vi "Create1.vi"(8 "error in (no error)":errorcluster) -> (0 "error out":errorcluster, 2 "Model":refnum<class "3D Object.lvclass">, 3 "Level out":refnum<class "Level.lvclass">)   [LabVIEW 2015, in "Level.lvclass"]
uses:
  Level.lvclass
  3D Object/3D Object.lvclass
  Segment.ctl
  Point.ctl
  Level.lvclass/Level.ctl
  3D Object/Object.vi
  3D Object/Box.vi
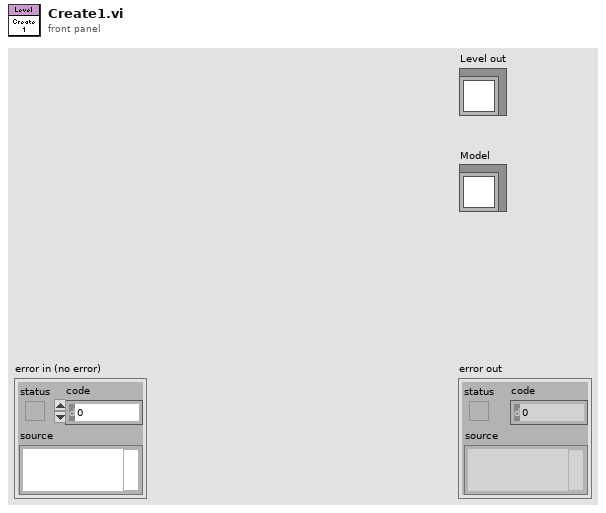
[diagram p1: front panel]
types:
  T1 = enum16{"As a Decal", "With Modulation", "With Blending", "As a replacement"}
  T2 = enum16{"No Filtration", "Linear Filtration", "Simple Mipmap Filtration", "Bilinear Filtration", "Trilinear Filtration"}
  T3 = cluster{"MinX":sgl, "MaxX":sgl, "MinZ":sgl, "MaxZ":sgl, "MinY":sgl, "MaxY":sgl}
  T4 = cluster{"Length X":sgl, "Length Y":sgl, "Length Z":sgl}
  T5 = typedef "Level.lvclass/Segment.ctl" = cluster{"Point 1":T6, "Point 2":T6}
  T6 = typedef "Level.lvclass/Point.ctl" = cluster{"Z":dbl, "X":dbl}
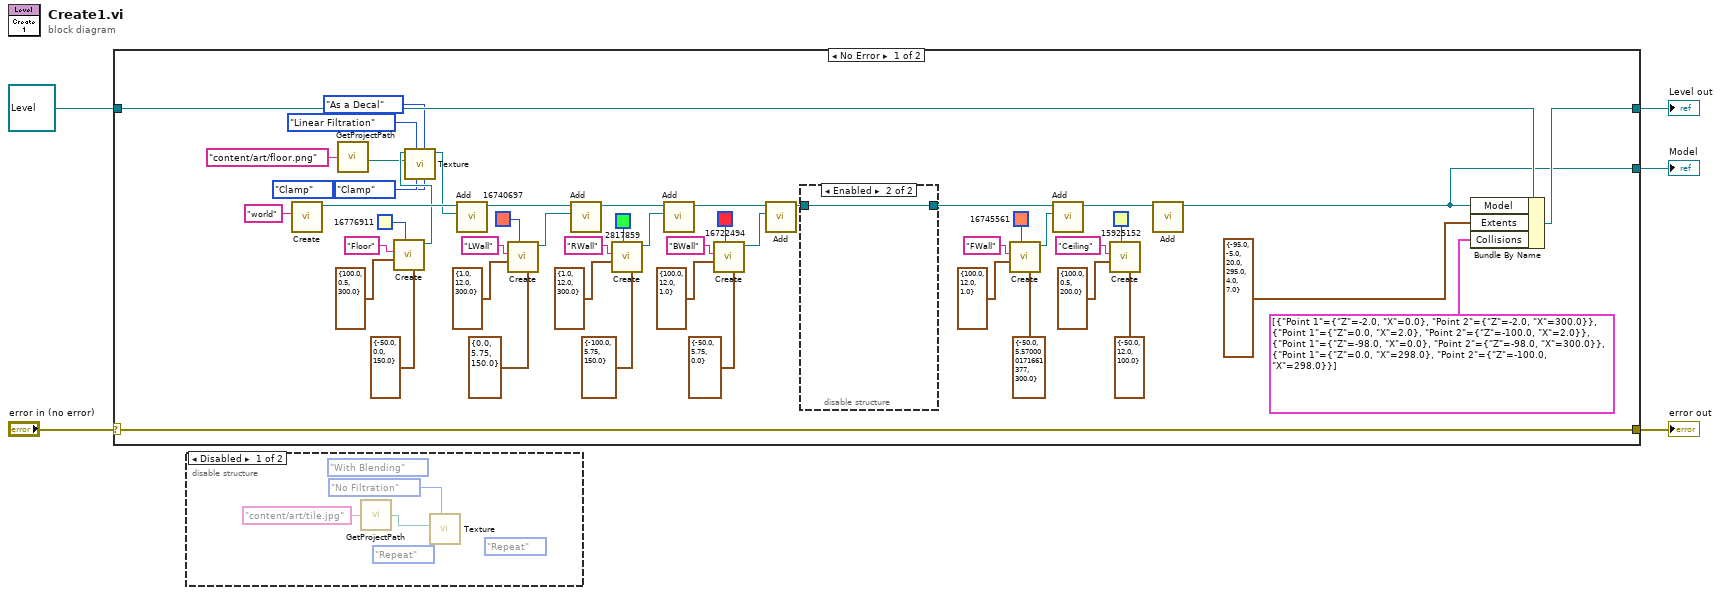
[diagram p0: block diagram]
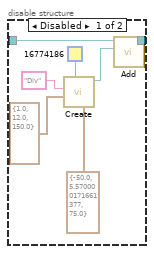
[diagram p3: hidden frame]
diagram:
  n1 = case shown="No Error" "error in (no error)" {
    selector: "error in (no error)" -> [w55 w65]
    tunnel: [w55 w65] -> w4
    tunnel: [w51 w64] -> w2
    tunnel: refnum<class "Level.lvclass"> refnum ("Level in") -> [w52 w64]
    tunnel: [w16 _] -> w1
    frame No Error {
      n2 = call-poly "Create.vi"("Name"="world") -> ("3D Object out"=w17:refnum<class "3D Object.lvclass">)  [unwired: 9 in, 1 out]
      n3 = call "GetProjectPath.vi"("File"="content/art/floor.png") -> ("Path"=w14:path)
      n4 = call-poly "Create.vi"("Position"=cluster{"X":sgl, "Y":sgl, "Z":sgl} {"X"=-50.0, "Y"=0.0, "Z"=150.0}, "Color Box"=u32 16776911, "Size"=T4 {"Length X"=100.0, "Length Y"=0.5, "Length Z"=300.0}, "Name"="Floor") -> ("3D Object out"=w15:refnum<class "3D Object.lvclass">)  [unwired: 6 in, 1 out]
      n5 = call "Texture.vi"("Vertical Wrap Mode"=enum16{"Clamp", "Repeat"}."Clamp", "Apply Mode"=T1."As a Decal", "Horizontal Wrap Mode"=enum16{"Clamp", "Repeat"}."Clamp", "Filter Mode"=T2."Linear Filtration", "path to image"=w14, "Object in"=w15) -> ("Object out"=w8:refnum<class "3D Object.lvclass">)  [unwired: 4 in, 1 out]
      n6 = call "Add.vi"("Child in"=w8, "Parent in"=w17) -> ("Parent out"=w18:refnum<class "3D Object.lvclass">)  [unwired: 7 in, 2 out]
      n7 = call-poly "Create.vi"("Position"=cluster{"X":sgl, "Y":sgl, "Z":sgl} {"X"=0.0, "Y"=5.75, "Z"=150.0}, "Color Box"=u32 16740697, "Size"=T4 {"Length X"=1.0, "Length Y"=12.0, "Length Z"=300.0}, "Name"="LWall") -> ("3D Object out"=w45:refnum<class "3D Object.lvclass">)  [unwired: 6 in, 1 out]
      n8 = call "Add.vi"("Child in"=w45, "Parent in"=w18) -> ("Parent out"=w44:refnum<class "3D Object.lvclass">)  [unwired: 7 in, 2 out]
      n9 = call-poly "Create.vi"("Position"=cluster{"X":sgl, "Y":sgl, "Z":sgl} {"X"=-100.0, "Y"=5.75, "Z"=150.0}, "Color Box"=u32 2817859, "Size"=T4 {"Length X"=1.0, "Length Y"=12.0, "Length Z"=300.0}, "Name"="RWall") -> ("3D Object out"=w43:refnum<class "3D Object.lvclass">)  [unwired: 6 in, 1 out]
      n10 = call "Add.vi"("Child in"=w43, "Parent in"=w44) -> ("Parent out"=w40:refnum<class "3D Object.lvclass">)  [unwired: 7 in, 2 out]
      n11 = call-poly "Create.vi"("Position"=cluster{"X":sgl, "Y":sgl, "Z":sgl} {"X"=-50.0, "Y"=5.75, "Z"=0.0}, "Color Box"=u32 16722494, "Size"=T4 {"Length X"=100.0, "Length Y"=12.0, "Length Z"=1.0}, "Name"="BWall") -> ("3D Object out"=w7:refnum<class "3D Object.lvclass">)  [unwired: 6 in, 1 out]
      n12 = call "Add.vi"("Child in"=w7, "Parent in"=w40) -> ("Parent out"=w34:refnum<class "3D Object.lvclass">)  [unwired: 7 in, 2 out]
      n13 = disable-structure shown="Enabled" {
        disable-tunnel: w34 -> [w62 w63]
        disable-tunnel: [w57 w63] -> w27
        frame Disabled {
          n14 = call-poly "Create.vi"("Position"=cluster{"X":sgl, "Y":sgl, "Z":sgl} {"X"=-50.0, "Y"=5.57, "Z"=75.0}, "Color Box"=u32 16774186, "Size"=T4 {"Length X"=1.0, "Length Y"=12.0, "Length Z"=150.0}, "Name"="Div") -> ("3D Object out"=w61:refnum<class "3D Object.lvclass">)  [unwired: 6 in, 1 out]
          n15 = call "Add.vi"("Child in"=w61, "Parent in"=w62) -> ("Parent out"=w57:refnum<class "3D Object.lvclass">)  [unwired: 7 in, 2 out]
        }
        frame Enabled {
        }
      }
      n16 = call-poly "Create.vi"("Position"=cluster{"X":sgl, "Y":sgl, "Z":sgl} {"X"=-50.0, "Y"=5.57, "Z"=300.0}, "Color Box"=u32 16745561, "Size"=T4 {"Length X"=100.0, "Length Y"=12.0, "Length Z"=1.0}, "Name"="FWall") -> ("3D Object out"=w6:refnum<class "3D Object.lvclass">)  [unwired: 6 in, 1 out]
      n17 = call "Add.vi"("Child in"=w6, "Parent in"=w27) -> ("Parent out"=w26:refnum<class "3D Object.lvclass">)  [unwired: 7 in, 2 out]
      n18 = call-poly "Create.vi"("Position"=cluster{"X":sgl, "Y":sgl, "Z":sgl} {"X"=-50.0, "Y"=12.0, "Z"=100.0}, "Color Box"=u32 15925152, "Size"=T4 {"Length X"=100.0, "Length Y"=0.5, "Length Z"=200.0}, "Name"="Ceiling") -> ()  [unwired: 6 in, 2 out]
      n19 = call "Add.vi"("Parent in"=w26) -> ("Parent out"=w16:refnum<class "3D Object.lvclass">)  [unwired: 8 in, 2 out]
      n20 = Bundle By Name(cluster=w52, "Model"=w16, "Extents"=T3 {"MinX"=-95.0, "MaxX"=-5.0, "MinZ"=20.0, "MaxZ"=295.0, "MinY"=4.0, "MaxY"=7.0}, "Collisions"=T5[] [{"Point 1"={"Z"=-2.0, "X"=0.0}, "Point 2"={"Z"=-2.0, "X"=300.0}}, {"Point 1"={"Z"=0.0, "X"=2.0}, "Point 2"={"Z"=-100.0, "X"=2.0}}, {"Point 1"={"Z"=-98.0, "X"=0.0}, "Point 2"={"Z"=-98.0, "X"=300.0}}, {"Point 1"={"Z"=0.0, "X"=298.0}, "Point 2"={"Z"=-100.0, "X"=298.0}}]) -> (w51:refnum<class "Level.lvclass">)
    }
    frame Error {
    }
  }
  "error out" <- w4
  "Level out" <- w2
  "Model" <- w1
  n21 = disable-structure shown="Disabled" {
    frame Disabled {
      (unwired) enum16{"Clamp", "Repeat"}."Repeat" ("Vertical Wrap Mode")
      (unwired) enum16{"Clamp", "Repeat"}."Repeat" ("Horizontal Wrap Mode")
      (unwired) T1."With Blending" ("Apply Mode")
      n22 = call "GetProjectPath.vi"("File"="content/art/tile.jpg") -> ("Path"=w67:path)
      n23 = call "Texture.vi"("Filter Mode"=T2."No Filtration", "path to image"=w67) -> ()  [unwired: 8 in, 2 out]
    }
    frame Enabled {
    }
  }
